vi "Enqueue.vi"(8 "error in (no error)":errorcluster, 9 "Priority Number":i32, 10 "Element":variant, 11 "PriorityQueue in":refnum<class "PriorityQueue.lvclass">) -> (0 "error out":errorcluster, 3 "PriorityQueue out":refnum<class "PriorityQueue.lvclass">)   [LabVIEW 2019, in "PriorityQueue.lvclass"]
doc: "Places an element on the priority queue at the correct position according to the specified priority number. The element will go after all elements on the queue with a higher priority or the same priority, and before all elements with a lower priority.\n\nIf the Priority Number input does not correspond to an existing priority level, the element is given the lowest existing priority and placed on the queue."
uses:
  PriorityQueue.lvclass
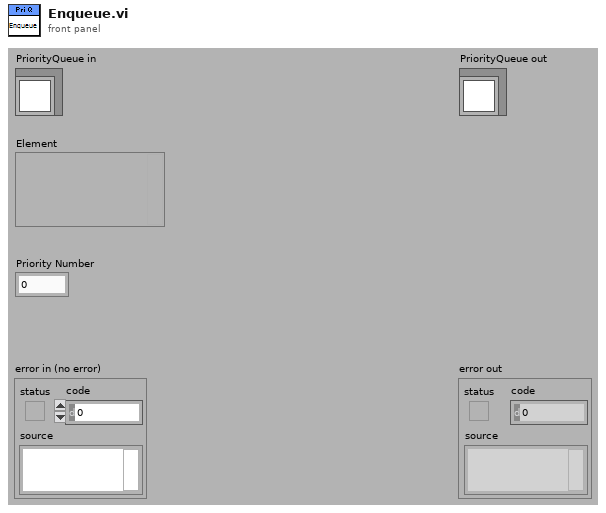
[diagram p1: front panel]
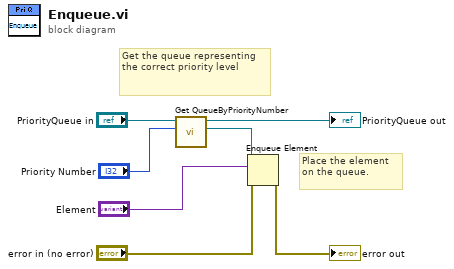
[diagram p0: block diagram]
diagram:
  # "Place the element on the queue."
  # "Get the queue representing the correct priority level"
  n1 = call "Get QueueByPriorityNumber.vi"("Priority Number"="Priority Number", "PriorityQueue in"="PriorityQueue in") -> ("Internal Queue"=w4:refnum<queue>, "PriorityQueue out"=→"PriorityQueue out":refnum<class "PriorityQueue.lvclass">)  [unwired: 7 in, 1 out]
  n2 = Enqueue Element(queue=w4, element="Element", error in (no error)="error in (no error)") -> (error out=→"error out":errorcluster)  [unwired: 1 in, 2 out]
